vi "ForceAndTubePressure.vi"() -> ()   [LabVIEW 2011]
uses:
  queue_driver/Control.ctl
  queue_driver/statesForcePressureExperiment.ctl
  <vilib>/DAQmx/read.llb/DAQmx Read (Analog DBL 1Chan 1Samp).vi
  <vilib>/DAQmx/read.llb/DAQmx Read (Analog 1D DBL NChan 1Samp).vi
  <vilib>/DAQmx/create/channels.llb/DAQmx Create Channel (AI-Voltage-Basic).vi
  <vilib>/DAQmx/miscellaneous.llb/DAQmx Fill In Error Info.vi
panel:
  out "standard error":string
  out "standard output":string
  out "Data file:":path
  out "Experiment Parameters file:":path
  out "Force":cluster{dbl, dbl}[](graph)
  out "voltage force":dbl
  out "pressure":dbl
  out "number":u32
  in  "Infusion Parameters":T1 {"Syringe - Volume (mL)" items=["5", "10", "20", "50"]; "Syringe - Make" items=["BBRAUN", "DISPOVAN", "BDINDIA"]}
  in  "Exit":bool
  in  "Capture":bool
  in  "Pressure Gauge Parameters":T2={"VISA resource name"="COM4", "Baud rate"=2400, "Data bits"=8, "Parity"=2, "Stop bits"=10, "Flow control"=0, "Sampling rate (Hz)"=1.0, "P gauge"="APG", "CE Channel"=""} {"Flow control" items=["None", "XON/XOFF", "RTS/CTS", "XON/XOFF & RTS/CTS", "DTR/DSR", "XON/XOFF & DTR/DSR"]; "Stop bits" items=["1.0"=10, "1.5"=15, "2.0"=20]; "Parity" items=["None", "Odd", "Even", "Mark", "Space"]; "Data bits" min=5 max=8 step=1}
  in  "Force Sensor Parameters":T3={"Sensor:"=0, "Sampling rate (Hz)"=100.0, "Sensor ID"="", "channels"=""} {"Sensor:" items=["FSG10WNPB", "FSG15WNPB", "ESS301", "A201", "Interlink-FSR", "Sensitronics-FSR"]}
  out "Pressure":cluster{dbl, dbl}[](graph)
  # "FORCE SENSOR - DYNAMIC TEST"
  # "version 2.0"
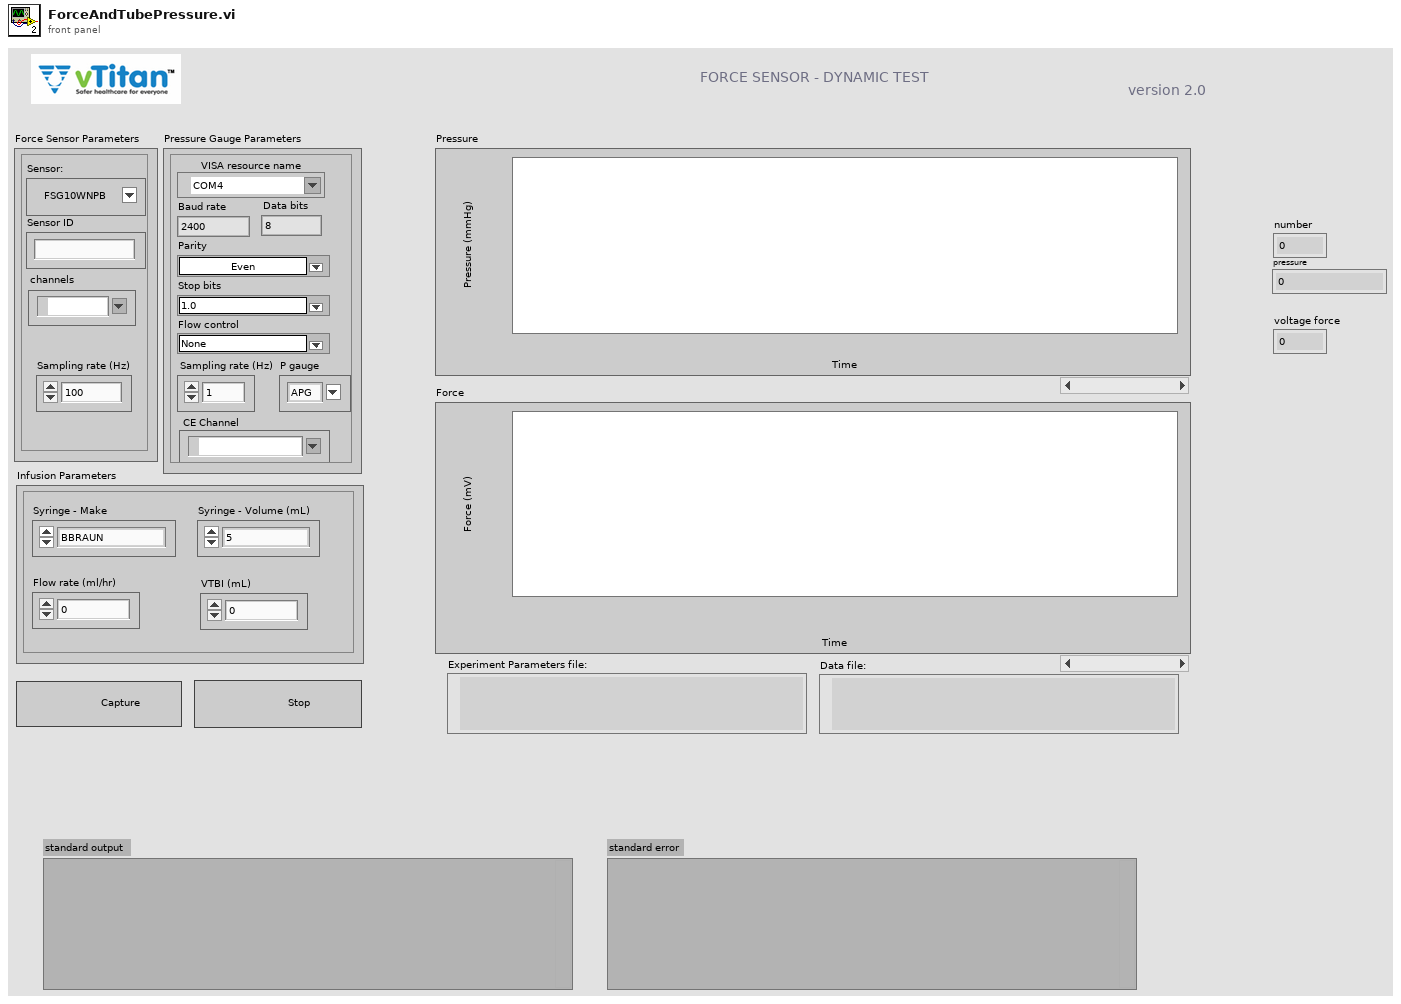
[diagram p1: front panel]
types:
  T1 = cluster{"Syringe - Make":u16, "Syringe - Volume (mL)":u16, "Flow rate (ml/hr)":dbl, "VTBI (mL)":dbl}
  T2 = cluster{"VISA resource name":refnum<visa-resource-name>, "Baud rate":u32, "Data bits":u16, "Parity":u16, "Stop bits":u16, "Flow control":u16, "Sampling rate (Hz)":dbl, "P gauge":string, "CE Channel":tag}
  T3 = cluster{"Sensor:":u16, "Sampling rate (Hz)":dbl, "Sensor ID":string, "channels":tag}
  T4 = cluster{"serial_refnum":refnum<visa-resource-name>, "daq_refnum":refnum<k21>, "log_file":path, "data_file":path, "force_sample_time":dbl, "pressure_sample_time":dbl, "last_force_sampled_time":u32, "last_pressure_sampled_time":u32, "start_capture":bool, "latest_pressure":dbl, "latest_force":dbl, "pressure_chart":cluster{dbl, "pressure":dbl}[], "force_chart":cluster{dbl, "pressure":dbl}[], "start_time":u32, "physical channels":tag, "CE Channel":tag, "CE_Refnum":refnum<k21>}
  T5 = typedef "statesForcePressureExperiment.ctl" = enum16{"Initialize", "Initialize-2", "write params log", "Poll", "Measure Pressure", "Measure Force", "run_script", "Exit"}
  T6 = typedef "Control.ctl" = enum16{"Create", "Enqueue-N", "Dequeue - 1 ", "Enstack - N", "Flush", "Release"}
  T7 = enum16{"open", "replace", "create", "open or create", "replace or create", "replace or create with confirmation"}
  T8 = enum32{"invalid app kind", "Development System", "Run Time System", "Student Edition", "Embedded LabVIEW", "Evaluation", "Custom"}
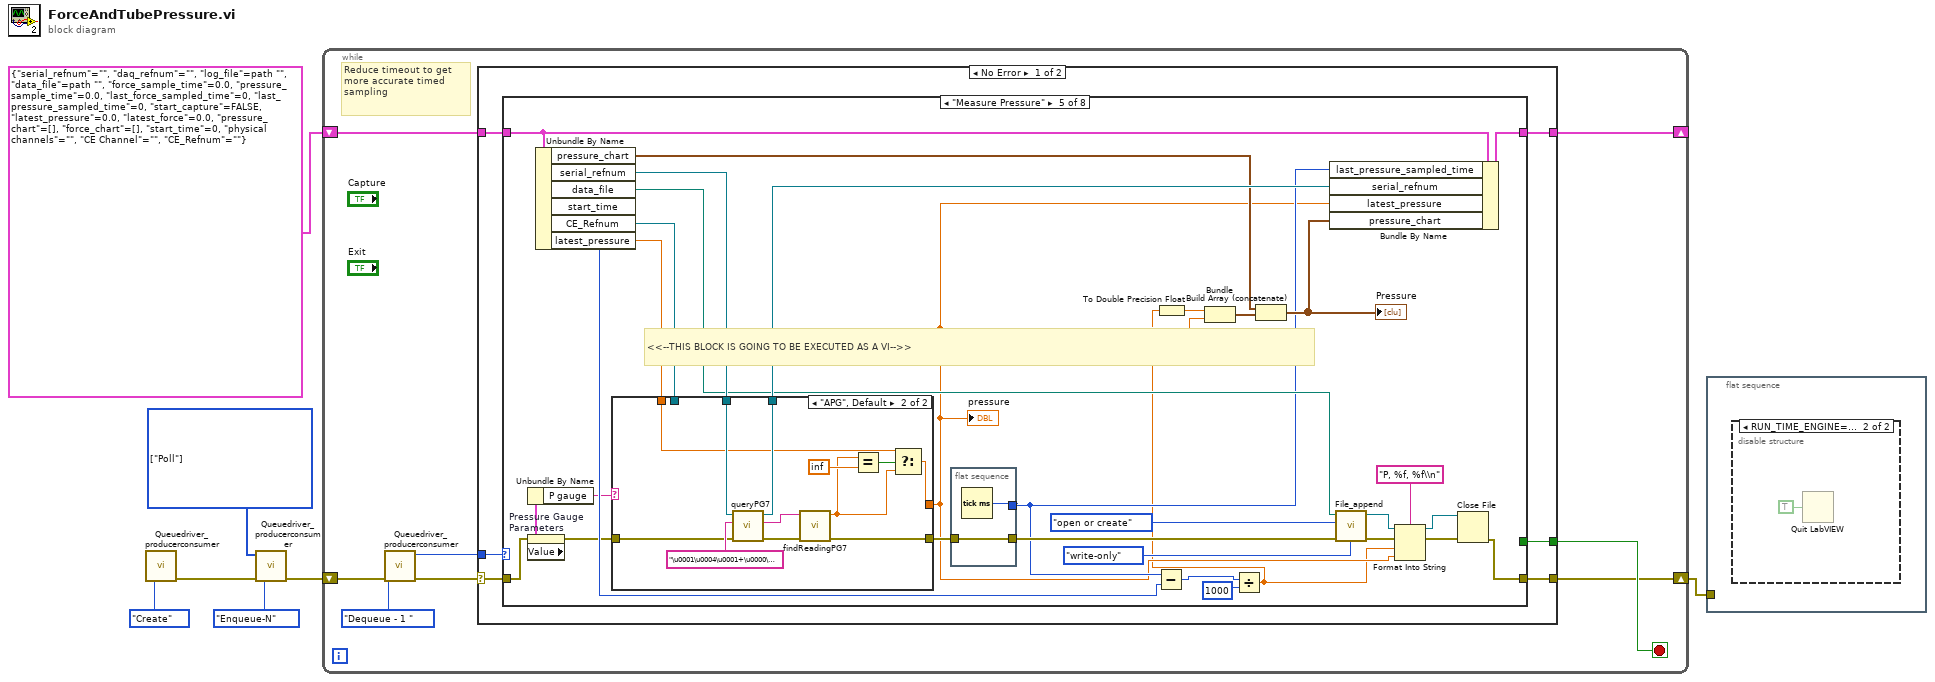
[diagram p0: block diagram]
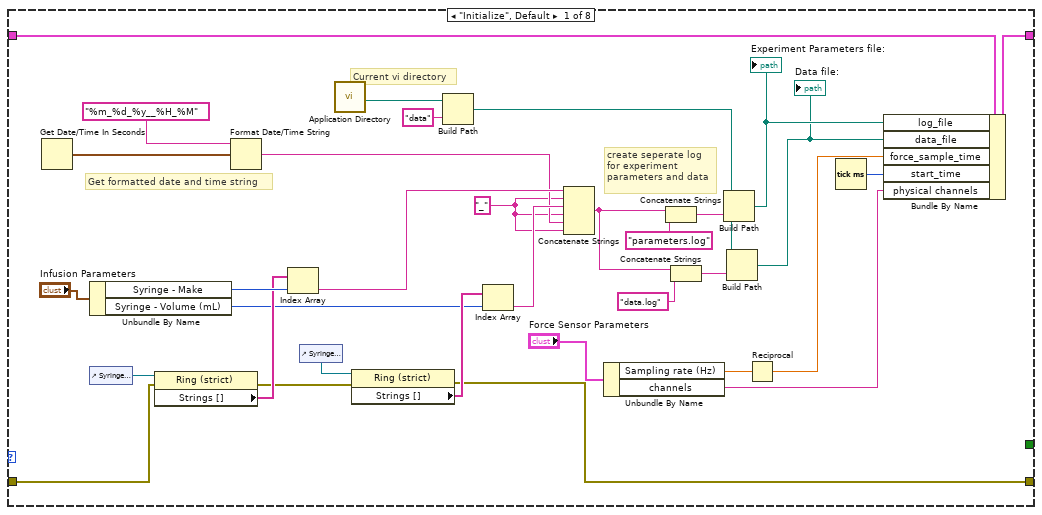
[diagram p3: hidden frame]
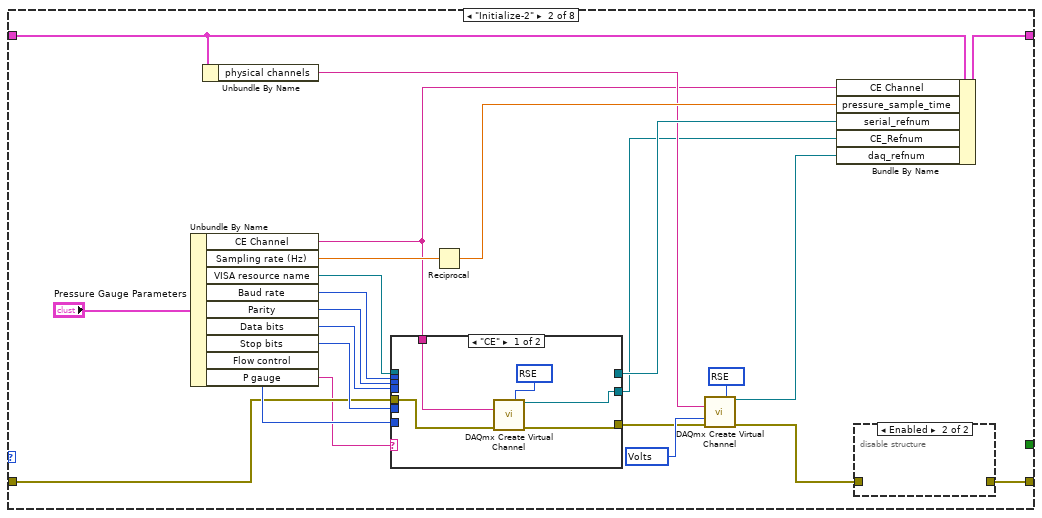
[diagram p4: hidden frame]
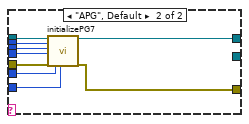
[diagram p5: hidden frame]
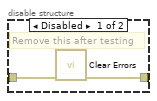
[diagram p6: hidden frame]
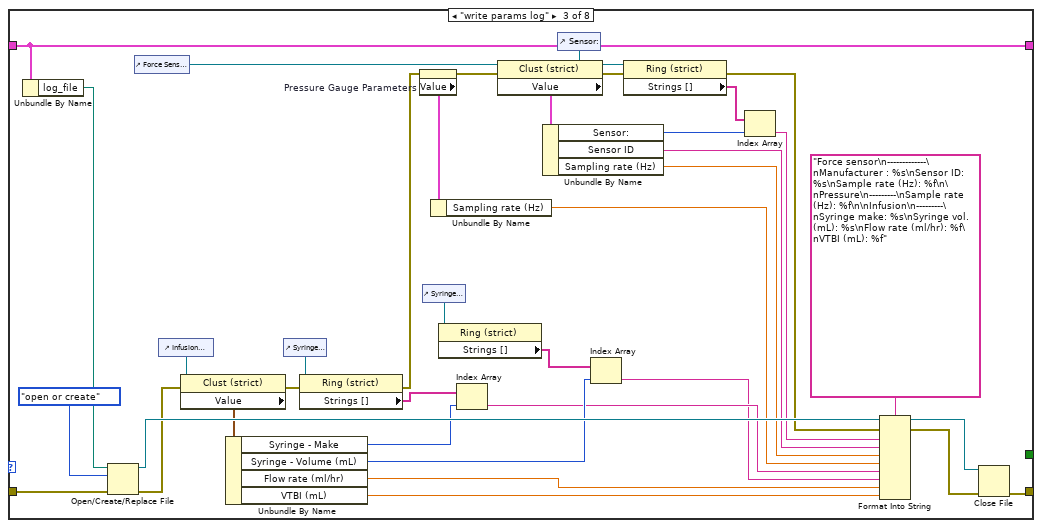
[diagram p7: hidden frame]
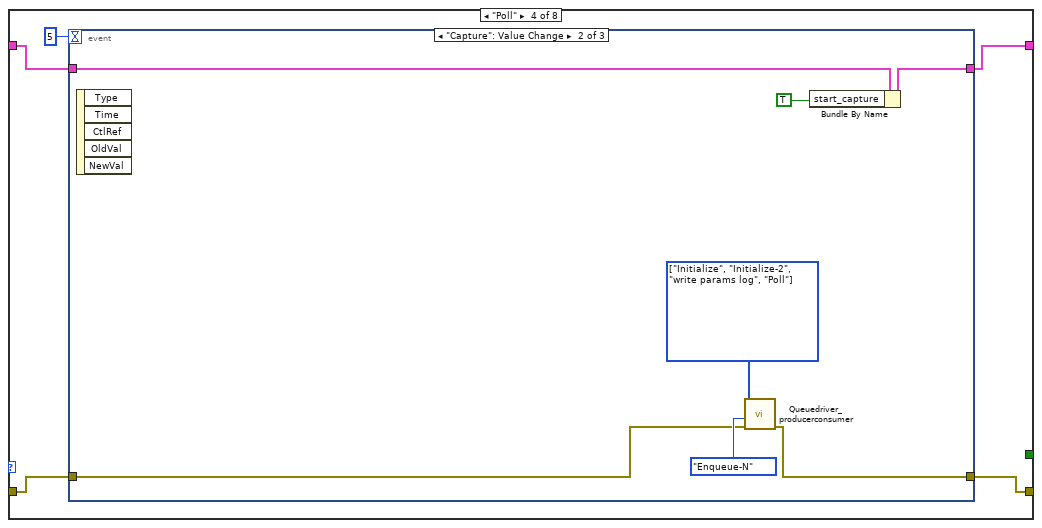
[diagram p8: hidden frame]
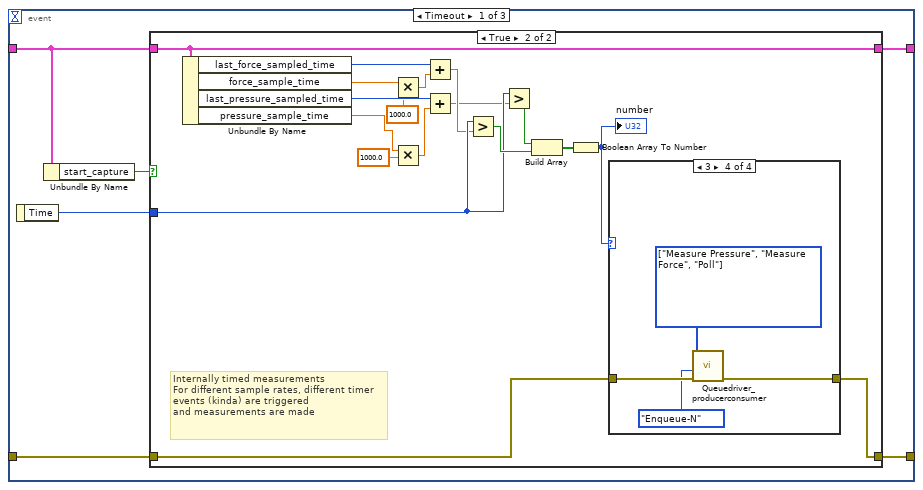
[diagram p9: hidden frame]
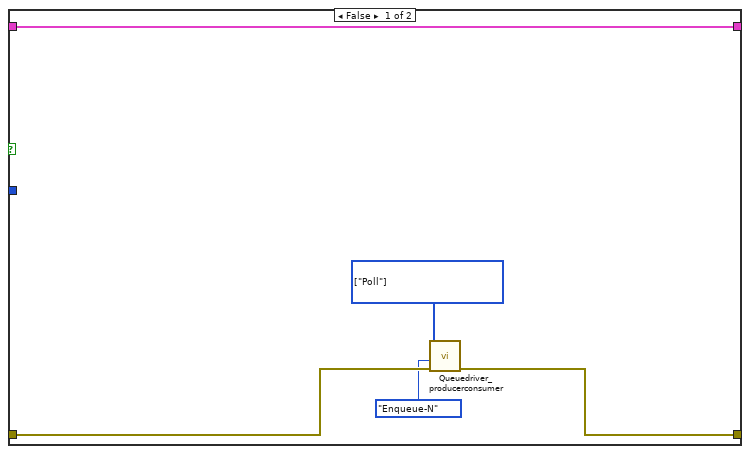
[diagram p10: hidden frame]
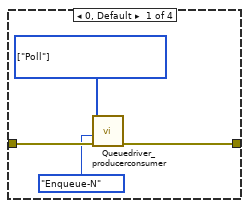
[diagram p11: hidden frame]
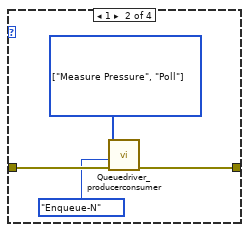
[diagram p12: hidden frame]
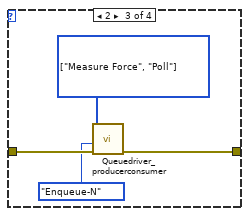
[diagram p13: hidden frame]
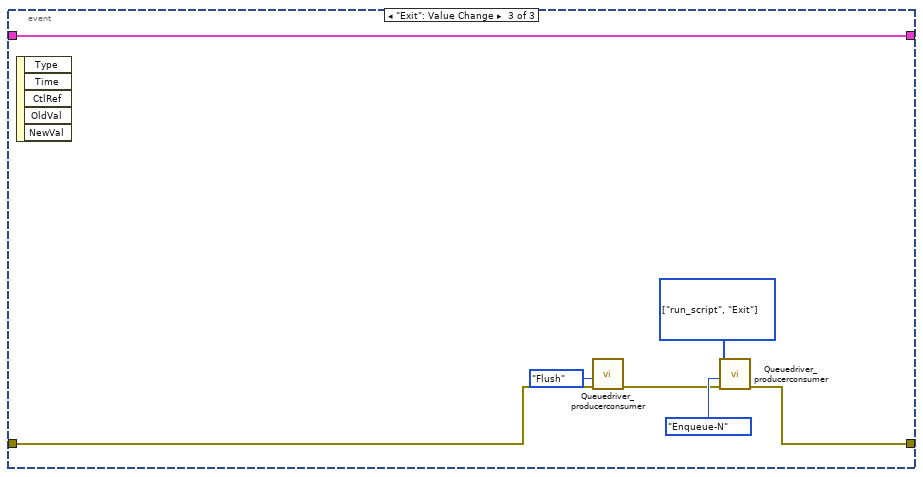
[diagram p14: hidden frame]
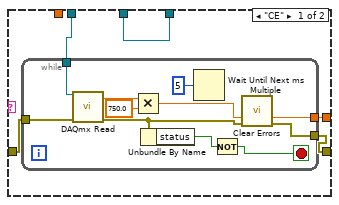
[diagram p15: hidden frame]
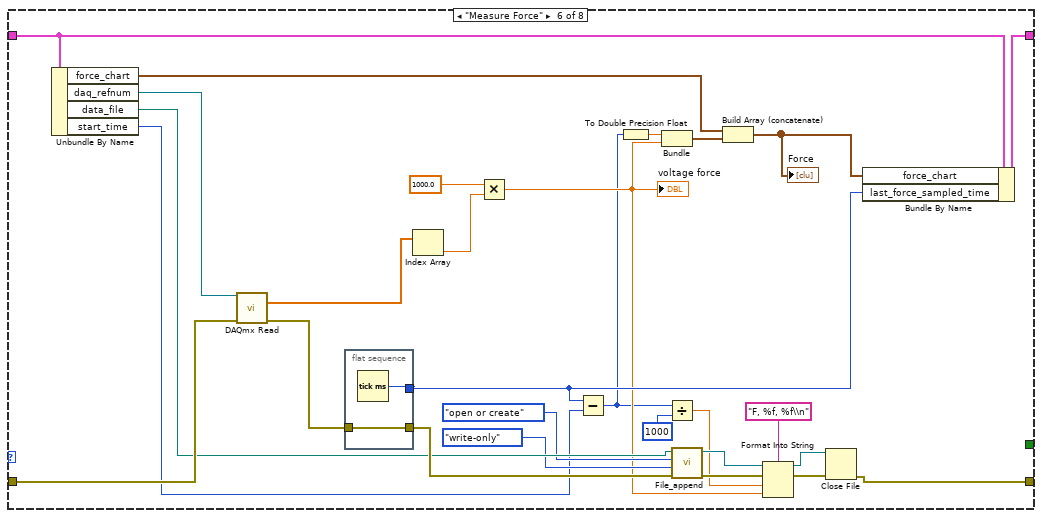
[diagram p16: hidden frame]
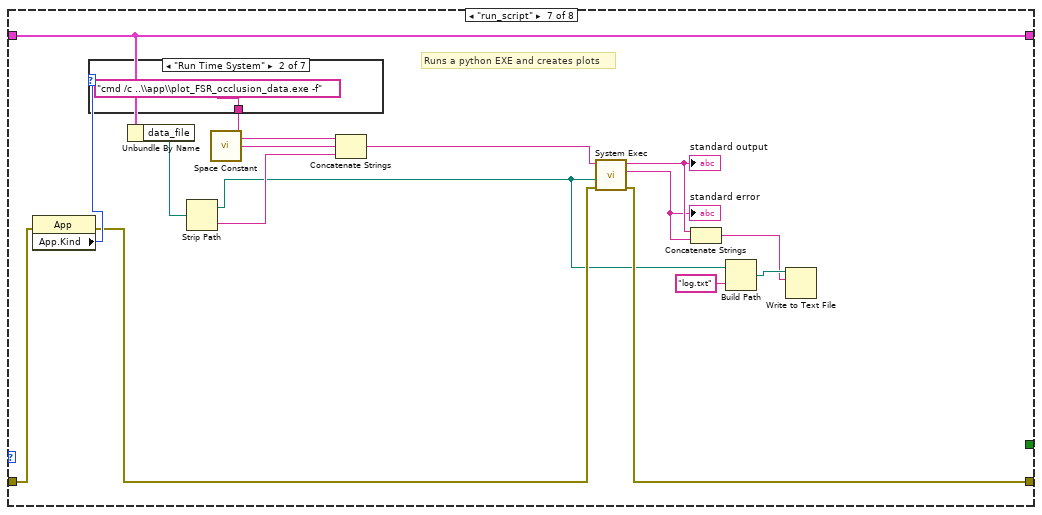
[diagram p17: hidden frame]
diagram:
  w3 = T5[] [enum."Poll"] items=["Initialize", "Initialize-2", "write params log", "Poll", "Measure Pressure", "Measure Force", "run_script", "Exit"] ("Enqueue")
  n1 = call "Queuedriver_producerconsumer.vi"("Operation"=Control."Create") -> ("error in 2"=w5:errorcluster)  [unwired: 9 in, 1 out]
  n2 = call "Queuedriver_producerconsumer.vi"("error in"=w5, "Operation"=Control."Enqueue-N", "Enqueue"=w3) -> ("error in 2"=w4:errorcluster)  [unwired: 7 in, 1 out]
  n3 = while {
    shift-right: [w9] -> w1
    shift-left: w4 -> [w15]
    shift-right: [w12] -> _
    shift-left: T4 {"serial_refnum"="", "daq_refnum"="", "log_file"=path "", "data_file"=path "", "force_sample_time"=0.0, "pressure_sample_time"=0.0, "last_force_sampled_time"=0, "last_pressure_sampled_time"=0, "start_capture"=FALSE, "latest_pressure"=0.0, "latest_force"=0.0, "pressure_chart"=[], "force_chart"=[], "start_time"=0, "physical channels"="", "CE Channel"="", "CE_Refnum"=""} -> [w13]
    stop <- w10 stop-if-true
    # "Reduce timeout to get more accurate timed sampling"
    n4 = call "Queuedriver_producerconsumer.vi"("error in"=w15, "Operation"=Control."Dequeue - 1 ") -> ("error in 2"=w8:errorcluster, "Dequeue"=w11:T5)  [unwired: 8 in]
    n5 = case shown="No Error" w8 {
      selector: w8 -> [w16 w312]
      tunnel: w13 -> [w21 w311]
      tunnel: [w20 w311] -> w12
      tunnel: w11 -> [w19 _]
      tunnel: [w18 FALSE] -> w10
      tunnel: [w17 w308] -> w9
      frame No Error {
        n6 = case shown="\"Measure Pressure\"" w19 {
          tunnel: w16 -> [w52 w70 w128 w135 w199 w272 w293 w305]
          tunnel: [w45 w67 w124 w134 w215 w259 w296 w305] -> w17
          tunnel: w21 -> [w38 w59 w130 w133 w223 w279 w300 w304]
          tunnel: [w37 w69 w130 w132 w222 w278 w300 w304] -> w20
          tunnel: [_ _ _ _ _ _ _ TRUE] -> w18
          frame "Initialize", Default {
            w39 = "_" ("string")
            # "create seperate log\nfor experiment\nparameters and data"
            # "Get formatted date and time string"
            # "Current vi directory"
            n7 = Get Date/Time In Seconds() -> (seconds since 1Jan1904=w42:timestamp)
            n8 = Unbundle By Name("Infusion Parameters") -> ("Syringe - Make"=w51:u16, "Syringe - Volume (mL)"=w46:u16)
            n9 = control-ref of="Syringe - Make"() -> (w53:refnum<vi>)
            n10 = property class="Ring (strict)"(reference=w53, error in=w52) -> (error out=w48:errorcluster, "Strings []"=w50:string[])  [unwired: 1 out]
            n11 = Format Date/Time String(time format string (%c)="%m_%d_%y__%H_%M", seconds (now)=w42) -> (date/time string=w40:string)  [unwired: 1 in]
            n12 = Index Array(array=w50, index=w51) -> (element=w44:string)
            n13 = control-ref of="Syringe - Volume (mL)"() -> (w49:refnum<vi>)
            n14 = call <vilib>:"Application Directory.vi"() -> ("Application Directory"=w22:path)
            n15 = property class="Ring (strict)"(reference=w49, error in=w48) -> (error out=w45:errorcluster, "Strings []"=w47:string[])  [unwired: 1 out]
            n16 = Build Path(base path=w22, name or relative path="data") -> (appended path=w30:path)
            n17 = Index Array(array=w47, index=w46) -> (element=w43:string)
            n18 = Concatenate Strings(w44, w39, w43, w39, w40, w39) -> (w31:string)
            n19 = Unbundle By Name("Force Sensor Parameters") -> ("Sampling rate (Hz)"=w26:dbl, "channels"=w23:tag)
            n20 = Concatenate Strings(w31, "parameters.log" ("string")) -> (w35:string)
            n21 = Concatenate Strings(w31, "data.log" ("string")) -> (w29:string)
            n22 = Build Path(base path=w30, name or relative path=w35) -> (appended path=w33:path)
            "Experiment Parameters file:" <- w33
            n23 = Build Path(base path=w30, name or relative path=w29) -> (appended path=w28:path)
            "Data file:" <- w28
            n24 = Reciprocal(x=w26) -> (1/x=w25:dbl)
            n25 = Tick Count (ms)() -> (millisecond timer value=w24:u32)
            n26 = Bundle By Name(cluster=w38, "log_file"=w33, "data_file"=w28, "force_sample_time"=w25, "start_time"=w24, "physical channels"=w23) -> (w37:T4)
          }
          frame "Initialize-2" {
            w63 = 10083 items=["default"=-1, "RSE"=10083, "NRSE"=10078, "Differential"=10106, "Pseudodifferential"=12529] ("input terminal configuration")
            w64 = 10348 items=["Volts"=10348, "From Custom Scale"=10065] ("units")
            n27 = Unbundle By Name("Pressure Gauge Parameters") -> ("CE Channel"=w55:tag, "Sampling rate (Hz)"=w66:dbl, "VISA resource name"=w77:refnum<visa-resource-name>, "Baud rate"=w76:u32, "Parity"=w75:u16, "Data bits"=w74:u16, "Stop bits"=w73:u16, "Flow control"=w72:u16, "P gauge"=w57:string)
            n28 = Unbundle By Name(w59) -> ("physical channels"=w58:tag)
            n29 = case shown="\"CE\"" w57 {
              tunnel: w77 -> [_ w91]
              tunnel: w76 -> [_ w90]
              tunnel: w75 -> [_ w89]
              tunnel: w74 -> [_ w88]
              tunnel: w73 -> [_ w87]
              tunnel: w72 -> [_ w86]
              tunnel: w70 -> [w81 w85]
              tunnel: [_ w84] -> w68
              tunnel: [w80 w83] -> w60
              tunnel: [w79 _] -> w56
              tunnel: w55 -> [w78 _]
              frame "CE" {
                w82 = 10083 items=["default"=-1, "RSE"=10083, "NRSE"=10078, "Differential"=10106, "Pseudodifferential"=12529] ("input terminal configuration")
                n30 = call-poly <vilib>:"DAQmx Create Virtual Channel.vi"("input terminal configuration"=w82, "physical channels"=w78, "error in"=w81) -> ("task out"=w79:refnum<k21>, "error out"=w80:errorcluster)  [unwired: 11 in]
              }
              frame "APG", Default {
                n31 = call "initializePG7.vi"("VISA resource name"=w91, "baud rate (9600)"=w90, "parity (0:none)"=w89, "data bits (8)"=w88, "error in (no error)"=w85, "stop bits (10: 1 bit)"=w87, "flow control (0:none)"=w86) -> ("VISA resource name 2"=w84:refnum<visa-resource-name>, "error IO"=w83:errorcluster)  [unwired: 11 in]
              }
            }
            n32 = Reciprocal(x=w66) -> (1/x=w65:dbl)
            n33 = call-poly <vilib>:"DAQmx Create Virtual Channel.vi"("input terminal configuration"=w63, "physical channels"=w58, "units"=w64, "error in"=w60) -> ("task out"=w61:refnum<k21>, "error out"=w62:errorcluster)  [unwired: 10 in]
            n34 = Bundle By Name(cluster=w59, "CE Channel"=w55, "pressure_sample_time"=w65, "serial_refnum"=w68, "CE_Refnum"=w56, "daq_refnum"=w61) -> (w69:T4)
            n35 = disable-structure shown="Enabled" {
              disable-tunnel: [w93 _] -> w67
              disable-tunnel: w62 -> [w92 _]
              frame Disabled {
                # "Remove this after testing"
                n36 = call <vilib>:"Clear Errors.vi"("error in (no error)"=w92) -> ("error out"=w93:errorcluster)  [unwired: 6 in]
              }
              frame Enabled {
              }
            }
          }
          frame "write params log" {
            n37 = Unbundle By Name(w130) -> ("log_file"=w129:path)
            n38 = Open/Create/Replace File(file path (use dialog)=w129, error in=w128, operation (0:open)=T7."open or create") -> (refnum out=w125:refnum<file>, error out=w119:errorcluster)  [unwired: 3 in, 1 out]
            n39 = control-ref of="Force Sensor Parameters"() -> (w118:refnum<vi>)
            n40 = control-ref of="Infusion Parameters"() -> (w121:refnum<vi>)
            n41 = property class="Clust (strict)"(reference=w121, error in=w119) -> (error out=w108:errorcluster, "Value"=w120:T1)  [unwired: 1 out]
            n42 = Unbundle By Name(w120) -> ("Syringe - Make"=w105:u16, "Syringe - Volume (mL)"=w102:u16, "Flow rate (ml/hr)"=w95:dbl, "VTBI (mL)"=w94:dbl)
            n43 = control-ref of="Syringe - Make"() -> (w115:refnum<vi>)
            n44 = property class="Ring (strict)"(reference=w115, error in=w108) -> (error out=w107:errorcluster, "Strings []"=w106:string[])  [unwired: 1 out]
            n45 = property on="Pressure Gauge Parameters" class="Clust (strict)"(error in=w107) -> (error out=w116:errorcluster, "Value"=w127:T2)  [unwired: 1 in, 1 out]
            n46 = control-ref of="Syringe - Volume (mL)"() -> (w104:refnum<vi>)
            n47 = Unbundle By Name(w127) -> ("Sampling rate (Hz)"=w100:dbl)
            n48 = property class="Ring (strict)"(reference=w104) -> ("Strings []"=w103:string[])  [unwired: 1 in, 2 out]
            n49 = Index Array(array=w106, index=w105) -> (element=w99:string)
            n50 = property class="Clust (strict)"(reference=w118, error in=w116) -> (error out=w111:errorcluster, "Value"=w117:T3)  [unwired: 1 out]
            n51 = Unbundle By Name(w117) -> ("Sensor:"=w112:u16, "Sensor ID"=w97:string, "Sampling rate (Hz)"=w96:dbl)
            n52 = control-ref of="Sensor:"() -> (w114:refnum<vi>)
            n53 = Index Array(array=w103, index=w102) -> (element=w98:string)
            n54 = property class="Ring (strict)"(reference=w114, error in=w111) -> (error out=w110:errorcluster, "Strings []"=w113:string[])  [unwired: 1 out]
            n55 = Index Array(array=w113, index=w112) -> (element=w109:string)
            n56 = Format Into String(format string="Force sensor\n-------------\nManufacturer : %s\nSensor ID: %s\nSample rate (Hz): %f\n\nPressure\n---------\nSample rate (Hz): %f\n\nInfusion\n---------\nSyringe make: %s\nSyringe vol. (mL): %s\nFlow rate (ml/hr): %f\nVTBI (mL): %f", initial string=w125, error in=w110, w109, w97, w96, w100, w99, w98, w95, w94) -> (resulting string=w123:refnum<file>, error out=w122:errorcluster)
            n57 = Close File(refnum=w123, error in=w122) -> (error out=w124:errorcluster)  [unwired: 1 out]
          }
          frame "Poll" {
            n58 = event shown="[1] \"Capture\": Value Change" {
              selector: _ -> [_ _ _]
              dyn-events: _ -> [_ _ _]
              timeout: 5 -> [_ _ _]
              tunnel: w135 -> [w141 w182 w191]
              tunnel: [w140 w181 w190] -> w134
              tunnel: w133 -> [w137 w187 w188]
              tunnel: [w138 w186 w188] -> w132
              event Timeout {
                n59 = event-data() -> ("Time"=w139:u32)  [unwired: 1 in]
                n60 = Unbundle By Name(w137) -> ("start_capture"=w136:bool)
                n61 = case shown="True" w136 {
                  tunnel: w141 -> [w145 w164]
                  tunnel: [w144 w163] -> w140
                  tunnel: w139 -> [_ w158]
                  tunnel: w137 -> [w146 w147]
                  tunnel: [w146 w147] -> w138
                  frame False {
                    w143 = T5[] [enum."Poll"] items=["Initialize", "Initialize-2", "write params log", "Poll", "Measure Pressure", "Measure Force", "run_script", "Exit"] ("Enqueue")
                    n62 = call "Queuedriver_producerconsumer.vi"("error in"=w145, "Operation"=Control."Enqueue-N", "Enqueue"=w143) -> ("error in 2"=w144:errorcluster)  [unwired: 7 in, 1 out]
                  }
                  frame True {
                    # "Internally timed measurements\nFor different sample rates, different timer events (kinda) are triggered\nand measurements are made"
                    n63 = Unbundle By Name(w147) -> ("last_force_sampled_time"=w156:u32, "force_sample_time"=w152:dbl, "last_pressure_sampled_time"=w157:u32, "pressure_sample_time"=w149:dbl)
                    n64 = Multiply(x=w152, y=1000.0) -> (x*y=w148:dbl)
                    n65 = Multiply(x=w149, y=1000.0) -> (x*y=w153:dbl)
                    n66 = Add(x=w156, y=w148) -> (x+y=w155:dbl)
                    n67 = Add(x=w157, y=w153) -> (x+y=w154:dbl)
                    n68 = Greater?(x=w158, y=w155) -> (0:w161:bool)
                    n69 = Greater?(x=w158, y=w154) -> (0:w162:bool)
                    n70 = Build Array(w162, w161) -> (w160:bool[])
                    n71 = Boolean Array To Number(Boolean array=w160) -> (number=w159:u32)
                    "number" <- w159
                    n72 = case shown="3" w159 {
                      tunnel: w164 -> [w167 w171 w175 w179]
                      tunnel: [w166 w170 w174 w178] -> w163
                      frame 0, Default {
                        w168 = T5[] [enum."Poll"] items=["Initialize", "Initialize-2", "write params log", "Poll", "Measure Pressure", "Measure Force", "run_script", "Exit"] ("Enqueue")
                        n73 = call "Queuedriver_producerconsumer.vi"("error in"=w167, "Operation"=Control."Enqueue-N", "Enqueue"=w168) -> ("error in 2"=w166:errorcluster)  [unwired: 7 in, 1 out]
                      }
                      frame 1 {
                        w172 = T5[] [enum."Measure Pressure", enum."Poll"] items=["Initialize", "Initialize-2", "write params log", "Poll", "Measure Pressure", "Measure Force", "run_script", "Exit"] ("Enqueue")
                        n74 = call "Queuedriver_producerconsumer.vi"("error in"=w171, "Operation"=Control."Enqueue-N", "Enqueue"=w172) -> ("error in 2"=w170:errorcluster)  [unwired: 7 in, 1 out]
                      }
                      frame 2 {
                        w176 = T5[] [enum."Measure Force", enum."Poll"] items=["Initialize", "Initialize-2", "write params log", "Poll", "Measure Pressure", "Measure Force", "run_script", "Exit"] ("Enqueue")
                        n75 = call "Queuedriver_producerconsumer.vi"("error in"=w175, "Operation"=Control."Enqueue-N", "Enqueue"=w176) -> ("error in 2"=w174:errorcluster)  [unwired: 7 in, 1 out]
                      }
                      frame 3 {
                        w180 = T5[] [enum."Measure Pressure", enum."Measure Force", enum."Poll"] items=["Initialize", "Initialize-2", "write params log", "Poll", "Measure Pressure", "Measure Force", "run_script", "Exit"] ("Enqueue")
                        n76 = call "Queuedriver_producerconsumer.vi"("error in"=w179, "Operation"=Control."Enqueue-N", "Enqueue"=w180) -> ("error in 2"=w178:errorcluster)  [unwired: 7 in, 1 out]
                      }
                    }
                  }
                }
              }
              event "Capture": Value Change {
                w184 = T5[] [enum."Initialize", enum."Initialize-2", enum."write params log", enum."Poll"] items=["Initialize", "Initialize-2", "write params log", "Poll", "Measure Pressure", "Measure Force", "run_script", "Exit"] ("Enqueue")
                n77 = event-data() -> ()  [unwired: 1 in, 5 out]
                n78 = call "Queuedriver_producerconsumer.vi"("error in"=w182, "Operation"=Control."Enqueue-N", "Enqueue"=w184) -> ("error in 2"=w181:errorcluster)  [unwired: 7 in, 1 out]
                n79 = Bundle By Name(cluster=w187, "start_capture"=TRUE) -> (w186:T4)
              }
              event "Exit": Value Change {
                w194 = T5[] [enum."run_script", enum."Exit"] items=["Initialize", "Initialize-2", "write params log", "Poll", "Measure Pressure", "Measure Force", "run_script", "Exit"] ("Enqueue")
                n80 = event-data() -> ()  [unwired: 1 in, 5 out]
                n81 = call "Queuedriver_producerconsumer.vi"("error in"=w191, "Operation"=Control."Flush") -> ("error in 2"=w192:errorcluster)  [unwired: 8 in, 1 out]
                n82 = call "Queuedriver_producerconsumer.vi"("error in"=w192, "Operation"=Control."Enqueue-N", "Enqueue"=w194) -> ("error in 2"=w190:errorcluster)  [unwired: 7 in, 1 out]
              }
            }
          }
          frame "Measure Pressure" {
            # "<<--THIS BLOCK IS GOING TO BE EXECUTED AS A VI-->>"
            n83 = property on="Pressure Gauge Parameters" class="Clust (strict)"(error in=w199) -> (error out=w198:errorcluster, "Value"=w200:T2)  [unwired: 1 in, 1 out]
            n84 = Unbundle By Name(w200) -> ("P gauge"=w197:string)
            n85 = Unbundle By Name(w223) -> ("pressure_chart"=w219:cluster{dbl, "pressure":dbl}[], "serial_refnum"=w224:refnum<visa-resource-name>, "data_file"=w214:path, "start_time"=w208:u32, "CE_Refnum"=w196:refnum<k21>, "latest_pressure"=w195:dbl)
            n86 = case shown="\"APG\", Default" w197 {
              tunnel: [w230 w249] -> w225
              tunnel: w224 -> [w230 w248]
              tunnel: [w229 w247] -> w217
              tunnel: [w228 w243] -> w205
              tunnel: w198 -> [w227 w246]
              tunnel: w196 -> [w226 _]
              tunnel: w195 -> [_ w241]
              frame "CE" {
                n87 = while {
                  tunnel: [w236] -> w229
                  tunnel: [w238] -> w228
                  tunnel: w227 -> [w232]
                  tunnel: w226 -> [w231]
                  stop <- w233 stop-if-true
                  n88 = call-poly <vilib>:"DAQmx Read.vi"("task/channels in"=w231, "error in"=w232) -> ("data"=w240:dbl, "error out"=w237:errorcluster)  [unwired: 11 in, 1 out]
                  n89 = Multiply(x=w240, y=750.0) -> (x*y=w238:dbl)
                  n90 = Unbundle By Name(w237) -> ("status"=w234:bool)
                  n91 = Wait Until Next ms Multiple(millisecond multiple=u32 5) -> ()  [unwired: 1 out]
                  n92 = Not(x=w234) -> (.not. x?=w233:bool)
                  n93 = call <vilib>:"Clear Errors.vi"("error in (no error)"=w237) -> ("error out"=w236:errorcluster)  [unwired: 6 in]
                }
              }
              frame "APG", Default {
                n94 = call "queryPG7.vi"("error in (no error)"=w246, "write buffer"="\u0001\u0004\u0001+\u0000\u0001@>", "VISA resource name"=w248) -> ("error IO"=w252:errorcluster, "read buffer"=w251:string, "VISA resource name 2"=w249:refnum<visa-resource-name>)  [unwired: 6 in]
                n95 = call "findReadingPG7.vi"("error in"=w252, "return string"=w251) -> ("error out"=w247:errorcluster, "pressure"=w242:dbl)  [unwired: 8 in]
                n96 = Equal?(x=w242, y=inf) -> (x = y?=w244:bool)
                n97 = Select(t=w241, s=w244, f=w242) -> (s? t:f=w243:dbl)
              }
            }
            "pressure" <- w205
            n98 = flat-sequence {
              tunnel: w217 -> [w254]
              tunnel: [w254] -> w216
              tunnel: [w253] -> w207
              frame #0 {
                n99 = Tick Count (ms)() -> (millisecond timer value=w253:u32)
              }
            }
            n100 = Subtract(x=w207, y=w208) -> (x-y=w202:u32)
            n101 = Divide(x=w202, y=u32 1000) -> (x/y=w201:dbl)
            n102 = To Double Precision Float(number=w201) -> (double precision float=w221:dbl)
            n103 = Bundle(w221, "pressure"=w205) -> (w220:cluster{dbl, "pressure":dbl})  [unwired: 1 in]
            n104 = Build Array (concatenate)(w219, w220) -> (w218:cluster{dbl, "pressure":dbl}[])
            "Pressure" <- w218
            n105 = Bundle By Name(cluster=w223, "last_pressure_sampled_time"=w207, "serial_refnum"=w225, "latest_pressure"=w205, "pressure_chart"=w218) -> (w222:T4)
            n106 = call "File_append.vi"("error in (no error)"=w216, "access (0:read/write)"=enum16{"read/write", "read-only", "write-only"}."write-only", "operation (0:open)"=T7."open or create", "data_file"=w214) -> ("error out"=w204:errorcluster, "Byte Stream File out"=w203:refnum<file>)  [unwired: 5 in, 1 out]
            n107 = Format Into String(format string="P, %f, %f\\n", initial string=w203, error in=w204, w201, w205) -> (resulting string=w210:refnum<file>, error out=w211:errorcluster)
            n108 = Close File(refnum=w210, error in=w211) -> (error out=w215:errorcluster)  [unwired: 1 out]
          }
          frame "Measure Force" {
            n109 = Unbundle By Name(w279) -> ("force_chart"=w274:cluster{dbl, "pressure":dbl}[], "daq_refnum"=w282:refnum<k21>, "data_file"=w265:path, "start_time"=w261:u32)
            n110 = call-poly <vilib>:"DAQmx Read.vi"("task/channels in"=w282, "error in"=w272) -> ("data"=w280:dbl[], "error out"=w273:errorcluster)  [unwired: 11 in, 1 out]
            n111 = flat-sequence {
              tunnel: [w284] -> w262
              tunnel: w273 -> [w283]
              tunnel: [w283] -> w266
              frame #0 {
                n112 = Tick Count (ms)() -> (millisecond timer value=w284:u32)
              }
            }
            n113 = Index Array(array=w280) -> (element=w277:dbl)  [unwired: 1 in]
            n114 = Multiply(x=1000.0, y=w277) -> (x*y=w260:dbl)
            "voltage force" <- w260
            n115 = Subtract(x=w262, y=w261) -> (x-y=w255:u32)
            n116 = To Double Precision Float(number=w255) -> (double precision float=w275:dbl)
            n117 = Bundle(w275, w260) -> (w276:cluster{dbl, dbl})  [unwired: 1 in]
            n118 = Divide(x=w255, y=u32 1000) -> (x/y=w257:dbl)
            n119 = call "File_append.vi"("error in (no error)"=w266, "access (0:read/write)"=enum16{"read/write", "read-only", "write-only"}."write-only", "operation (0:open)"=T7."open or create", "data_file"=w265) -> ("error out"=w268:errorcluster, "Byte Stream File out"=w267:refnum<file>)  [unwired: 5 in, 1 out]
            n120 = Build Array (concatenate)(w274, w276) -> (w256:cluster{dbl, "pressure":dbl}[])
            "Force" <- w256
            n121 = Format Into String(format string="F, %f, %f\\n", initial string=w267, error in=w268, w257, w260) -> (resulting string=w270:refnum<file>, error out=w271:errorcluster)
            n122 = Close File(refnum=w270, error in=w271) -> (error out=w259:errorcluster)  [unwired: 1 out]
            n123 = Bundle By Name(cluster=w279, "force_chart"=w256, "last_force_sampled_time"=w262) -> (w278:T4)
          }
          frame "run_script" {
            # "Runs a python EXE and creates plots"
            n124 = property class="App"(error in=w293) -> (error out=w292:errorcluster, "App.Kind"=w294:T8)  [unwired: 1 in, 1 out]
            n125 = case shown="\"Run Time System\"" w294 {
              tunnel: [_ "cmd /c ..\\app\\plot_FSR_occlusion_data.exe -f" ("string") _ _ _ _ "python ..\\scripts\\plot_FSR_occlusion_data.py -f" ("string")] -> w299
              frame "invalid app kind" {
              }
              frame "Run Time System" {
              }
              frame "Student Edition" {
              }
              frame "Embedded LabVIEW" {
              }
              frame "Evaluation" {
              }
              frame "Custom" {
              }
              frame "Development System" {
              }
            }
            n126 = Unbundle By Name(w300) -> ("data_file"=w291:path)
            n127 = Strip Path(path=w291) -> (stripped path=w289:path, name=w295:string)
            n128 = call <vilib>:"Space Constant.vi"() -> ("String"=w298:string)
            n129 = Concatenate Strings(w299, w298, w295) -> (w297:string)
            n130 = call <vilib>:"System Exec.vi"("error in (no error)"=w292, "working directory"=w289, "command line"=w297) -> ("error out"=w296:errorcluster, "standard error"=w286:string, "standard output"=w287:string)  [unwired: 5 in, 1 out]
            "standard output" <- w287
            "standard error" <- w286
            n131 = Concatenate Strings(w287, w286) -> (w285:string)
            n132 = Build Path(base path=w289, name or relative path="log.txt") -> (appended path=w290:path)
            n133 = Write to Text File(file (use dialog)=w290, text=w285) -> ()  [unwired: 2 in, 3 out]
          }
          frame "Exit" {
          }
        }
      }
      frame Error {
        w306 = T5[] [enum."Exit"] items=["Initialize", "Initialize-2", "write params log", "Poll", "Measure Pressure", "Measure Force", "run_script", "Exit"] ("Enqueue")
        n134 = call <vilib>:"Simple Error Handler.vi"("error in (no error)"=w312) -> ("error out"=w310:errorcluster)  [unwired: 4 in, 4 out]
        n135 = call <vilib>:"Clear Errors.vi"("error in (no error)"=w310) -> ("error out"=w309:errorcluster)  [unwired: 6 in]
        n136 = call "Queuedriver_producerconsumer.vi"("error in"=w309, "Operation"=Control."Enqueue-N", "Enqueue"=w306) -> ("error in 2"=w308:errorcluster)  [unwired: 7 in, 1 out]
      }
    }
  }
  n137 = flat-sequence {
    tunnel: w1 -> [_]
    frame #0 {
      n138 = disable-structure shown="RUN_TIME_ENGINE==True" {
        frame condition #0 (active) {
        }
        frame condition #1 {
          n139 = Quit LabVIEW(quit? (T)=TRUE) -> ()
        }
      }
    }
  }
